vi "OAT Tachless Mouse Pos to Eng Unit.vi"(2 "Pop Pos":cluster{i32, i32}, 3 "Tracks ref":refnum<vi>) -> (0 "Control Point":cluster{dbl, dbl} {"?" format="%.2f"; "?" format="%.2f"})   [LabVIEW 2017, in "SoundVib_Tachless.lvlib"]
uses:
  <vilib>/addons/Sound and Vibration/Order Analysis/Tachless/SoundVib_Tachless.lvlib
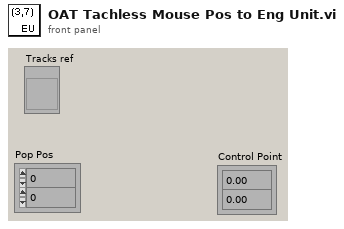
[diagram p1: front panel]
types:
  T1 = typedef "LVBoundsTypeDef.ctl" = cluster{"Width":u32, "Height":u32}
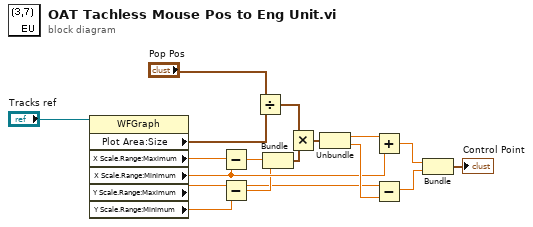
[diagram p0: block diagram]
diagram:
  n1 = property on="Property Node" class="WFGraph"(reference="Tracks ref") -> ("Plot Area:Size"=w6:T1, "X Scale.Range:Maximum"=w7:dbl, "X Scale.Range:Minimum"=w16:dbl, "Y Scale.Range:Maximum"=w8:dbl, "Y Scale.Range:Minimum"=w9:dbl)  [unwired: 1 in, 2 out]
  n2 = Subtract(x=w7, y=w16) -> (x-y=w10:dbl)
  n3 = Subtract(x=w8, y=w9) -> (x-y=w11:dbl)
  n4 = Divide(x="Pop Pos", y=w6) -> (x/y=w13:cluster{dbl, dbl})
  n5 = Bundle(w10, w11) -> (w12:cluster{dbl, dbl})  [unwired: 1 in]
  n6 = Multiply(x=w13, y=w12) -> (x*y=w14:cluster{dbl, dbl})
  n7 = Unbundle(w14) -> (w15:dbl, w17:dbl)
  n8 = Add(x=w15, y=w16) -> (x+y=w4:dbl)
  n9 = Subtract(x=w8, y=w17) -> (x-y=w3:dbl)
  n10 = Bundle(w4, w3) -> (→"Control Point":cluster{dbl, dbl})  [unwired: 1 in]
